vi "Load Functions from Disk.vi"(8 "error in (no error)":errorcluster, 10 "Array of paths (folders to scan or explicit files)":path[](array[path]), 11 "base path":path) -> (0 "error out":errorcluster, 2 "Available Functions":refnum<class "Function.lvclass">[](array[class]))   [LabVIEW 2016, in "Controller Actor.lvlib" / "Controller.lvclass"]
uses:
  <userlib>/Common Components/Controller/Controller.lvclass
  <userlib>/Common Components/Function Actor/Function.lvclass
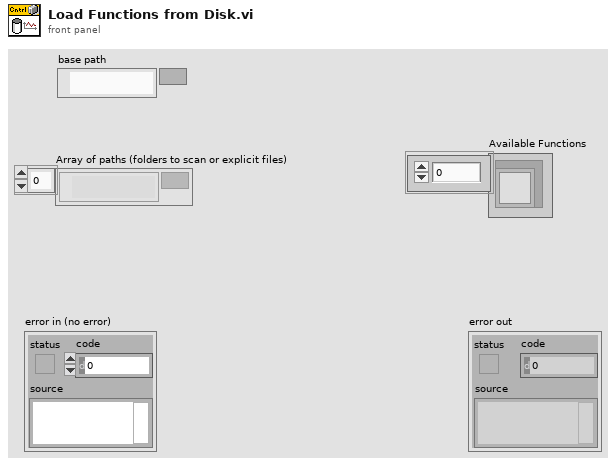
[diagram p1: front panel]
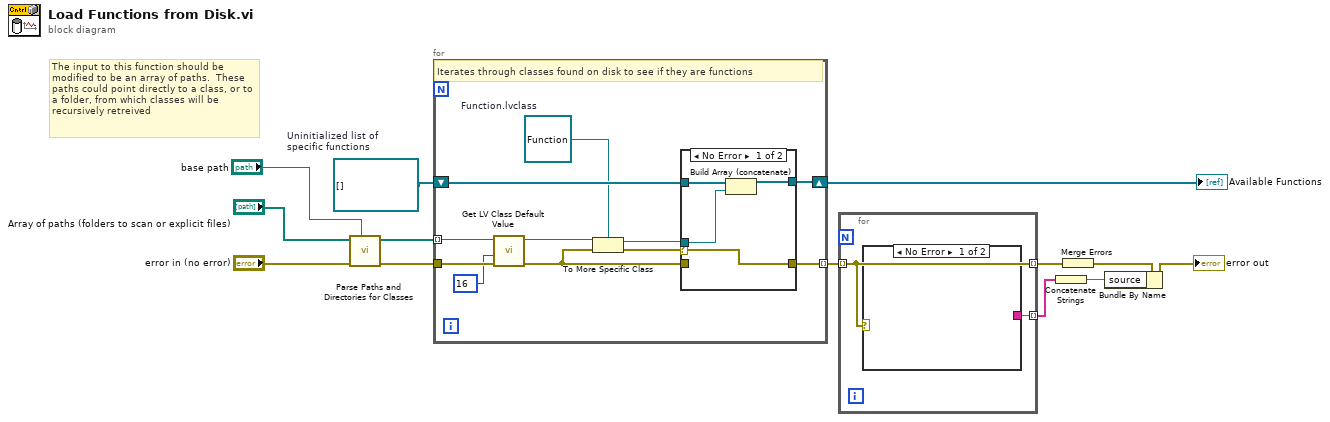
[diagram p0: block diagram]
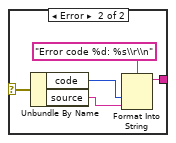
[diagram p2: hidden frame]
diagram:
  w13 = refnum<class "Function.lvclass">[] []  # Uninitialized list of specific functions
  # "The input to this function should be modified to be an array of paths.  These paths could point directly to a class, or to a folder, from which classes will be recursively retreived"
  n1 = call <userlib>:"Parse Paths and Directories for Classes.vi"("base path"="base path", "error in (no error)"="error in (no error)", "Array of paths (folders to scan or explicit files)"="Array of paths (folders to scan or explicit files)") -> ("error out"=w9:errorcluster, "All Files in Dir"=w10:path[])  [unwired: 7 in]
  n2 = for {
    shift-right: [w23] -> w12
    shift-left: w13 -> [w20]
    tunnel: w10 -> [w15] mode=indexing
    tunnel: w9 -> [w22]
    tunnel: [w21] -> w11 mode=indexing
    w18 = refnum<class "Function.lvclass"> refnum  # Function.lvclass
    # "Iterates through classes found on disk to see if they are functions"
    n3 = call <vilib>:"Get LV Class Default Value.vi"("error in (no error)"=w22, "options"=u32 16, "class path"=w15) -> ("error out"=w14:errorcluster, "object"=w19:refnum<class>)  [unwired: 7 in]
    n4 = To More Specific Class(target class=w18, reference=w19, error in=w14) -> (specific class reference=w24:refnum<class "Function.lvclass">, error out=w17:errorcluster)
    n5 = case shown="No Error" w17 {
      selector: w17 -> [w25 _]
      tunnel: w24 -> [w26 _]
      tunnel: [w28 w30] -> w23
      tunnel: w20 -> [w27 w30]
      tunnel: [w25 w29] -> w21
      tunnel: w14 -> [_ w29]
      frame No Error {
        n6 = Build Array (concatenate)(w27, w26) -> (w28:refnum<class "Function.lvclass">[])
      }
      frame Error {
      }
    }
  }
  "Available Functions" <- w12
  n7 = for {
    tunnel: w11 -> [w31] mode=indexing
    tunnel: [w32] -> w2 mode=indexing
    tunnel: [w31] -> w5 mode=indexing
    n8 = case shown="No Error" w31 {
      selector: w31 -> [_ w33]
      tunnel: [_ w34] -> w32
      frame No Error {
      }
      frame Error {
        n9 = Unbundle By Name(w33) -> ("code"=w36:i32, "source"=w35:string)
        n10 = Format Into String(format string="Error code %d: %s\\r\\n", w36, w35) -> (resulting string=w34:string)  [unwired: 2 in, 1 out]
      }
    }
  }
  n11 = Concatenate Strings(w2) -> (w1:string)
  n12 = Merge Errors(w5) -> (w4:errorcluster)
  n13 = Bundle By Name(cluster=w4, "source"=w1) -> (→"error out":errorcluster)
